vi "0 -5 Connect Message Display.vi"() -> ()   [LabVIEW 2012]
panel:
  out "Base + Entension Number":dbl
  in  "Base Number":dbl=1200.0 min=1000.0 step=10.0
  in  "OK Button":bool
  in  "Extension Number":dbl min=0.0 max=5.0 step=1.0
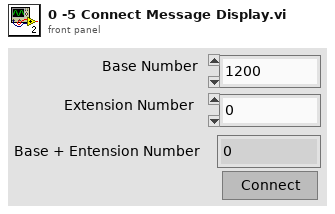
[diagram p1: front panel]
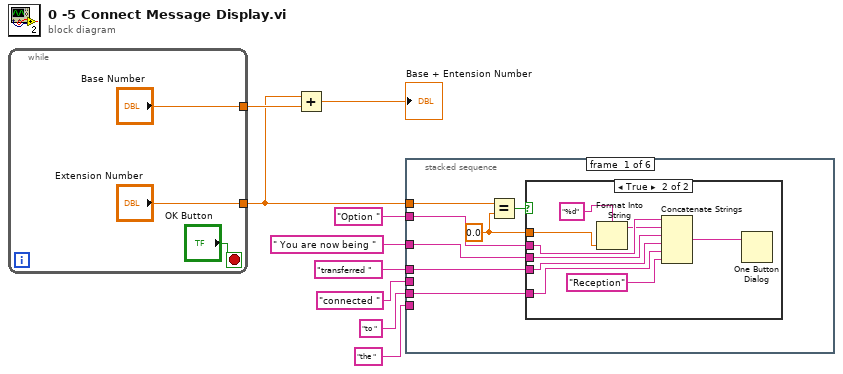
[diagram p0: block diagram]
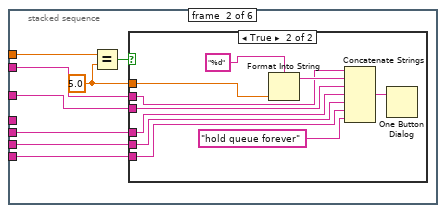
[diagram p3: hidden frame]
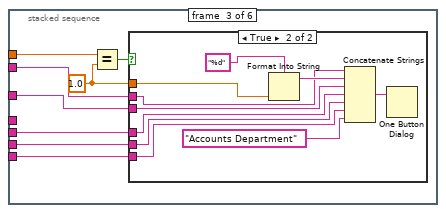
[diagram p5: hidden frame]
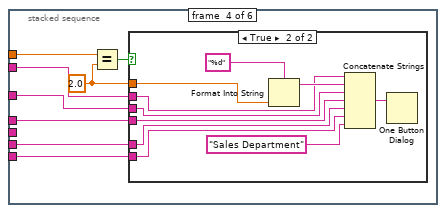
[diagram p7: hidden frame]
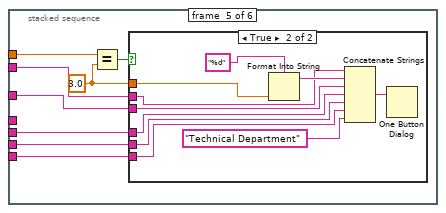
[diagram p9: hidden frame]
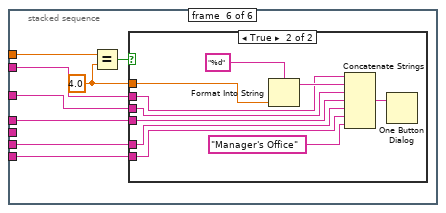
[diagram p11: hidden frame]
diagram:
  n1 = while {
    tunnel: ["Extension Number"] -> w1
    tunnel: ["Base Number"] -> w2
    stop <- "OK Button" stop-if-true
  }
  n2 = Add(x=w1, y=w2) -> (x+y=→"Base + Entension Number":dbl)
  n3 = stacked-sequence {
    tunnel: "Option " -> [w18 w30 w52 w70 w88 w105]
    tunnel: " You are now being " -> [w17 w31 w51 w69 w87 w104]
    tunnel: "transferred " -> [w16 _ _ w67 _ w103]
    tunnel: "to " -> [w15 w34 w49 w66 w83 w102]
    tunnel: w1 -> [w13 w29 w54 w68 w86 w106]
    tunnel: "connected " -> [_ w32 w50 _ w84 _]
    tunnel: "the " -> [_ w33 w48 w65 w85 w101]
    frame #0 {
      w14 = 0.0
      n4 = Equal?(x=w13, y=w14) -> (x = y?=w19:bool)
      n5 = case shown="True" w19 {
        tunnel: w18 -> [_ w28]
        tunnel: w17 -> [_ w26]
        tunnel: w16 -> [_ w25]
        tunnel: w15 -> [_ w24]
        tunnel: w14 -> [_ w22]
        frame False {
        }
        frame True {
          n6 = Format Into String(format string="%d", w22) -> (resulting string=w21:string)  [unwired: 2 in, 1 out]
          n7 = Concatenate Strings(w28, w21, w26, w25, w24, "Reception") -> (w27:string)
          n8 = One Button Dialog(message=w27) -> ()  [unwired: 1 in, 1 out]
        }
      }
    }
    frame #1 {
      w36 = 5.0
      n9 = Equal?(x=w29, y=w36) -> (x = y?=w35:bool)
      n10 = case shown="True" w35 {
        tunnel: w36 -> [_ w44]
        tunnel: w30 -> [_ w43]
        tunnel: w31 -> [_ w42]
        tunnel: w32 -> [_ w41]
        tunnel: w34 -> [_ w40]
        tunnel: w33 -> [_ w39]
        frame False {
        }
        frame True {
          n11 = Format Into String(format string="%d", w44) -> (resulting string=w45:string)  [unwired: 2 in, 1 out]
          n12 = Concatenate Strings(w43, w45, w42, w41, w40, w39, "hold queue forever") -> (w46:string)
          n13 = One Button Dialog(message=w46) -> ()  [unwired: 1 in, 1 out]
        }
      }
    }
    frame #2 {
      w53 = 1.0
      n14 = Equal?(x=w54, y=w53) -> (x = y?=w47:bool)
      n15 = case shown="True" w47 {
        tunnel: w53 -> [_ w62]
        tunnel: w52 -> [_ w61]
        tunnel: w51 -> [_ w60]
        tunnel: w50 -> [_ w59]
        tunnel: w49 -> [_ w58]
        tunnel: w48 -> [_ w57]
        frame False {
        }
        frame True {
          n16 = Format Into String(format string="%d", w62) -> (resulting string=w63:string)  [unwired: 2 in, 1 out]
          n17 = Concatenate Strings(w61, w63, w60, w59, w58, w57, "Accounts Department") -> (w64:string)
          n18 = One Button Dialog(message=w64) -> ()  [unwired: 1 in, 1 out]
        }
      }
    }
    frame #3 {
      w71 = 2.0
      n19 = Equal?(x=w68, y=w71) -> (x = y?=w72:bool)
      n20 = case shown="True" w72 {
        tunnel: w71 -> [_ w80]
        tunnel: w70 -> [_ w79]
        tunnel: w69 -> [_ w78]
        tunnel: w66 -> [_ w77]
        tunnel: w65 -> [_ w76]
        tunnel: w67 -> [_ w73]
        frame False {
        }
        frame True {
          n21 = Format Into String(format string="%d", w80) -> (resulting string=w81:string)  [unwired: 2 in, 1 out]
          n22 = Concatenate Strings(w79, w81, w78, w73, w77, w76, "Sales Department") -> (w82:string)
          n23 = One Button Dialog(message=w82) -> ()  [unwired: 1 in, 1 out]
        }
      }
    }
    frame #4 {
      w90 = 3.0
      n24 = Equal?(x=w86, y=w90) -> (x = y?=w89:bool)
      n25 = case shown="True" w89 {
        tunnel: w90 -> [_ w98]
        tunnel: w88 -> [_ w97]
        tunnel: w87 -> [_ w96]
        tunnel: w84 -> [_ w95]
        tunnel: w83 -> [_ w94]
        tunnel: w85 -> [_ w93]
        frame False {
        }
        frame True {
          n26 = Format Into String(format string="%d", w98) -> (resulting string=w99:string)  [unwired: 2 in, 1 out]
          n27 = Concatenate Strings(w97, w99, w96, w95, w94, w93, "Technical Department") -> (w100:string)
          n28 = One Button Dialog(message=w100) -> ()  [unwired: 1 in, 1 out]
        }
      }
    }
    frame #5 {
      w108 = 4.0
      n29 = Equal?(x=w106, y=w108) -> (x = y?=w107:bool)
      n30 = case shown="True" w107 {
        tunnel: w108 -> [_ w116]
        tunnel: w105 -> [_ w115]
        tunnel: w104 -> [_ w114]
        tunnel: w103 -> [_ w113]
        tunnel: w102 -> [_ w112]
        tunnel: w101 -> [_ w109]
        frame False {
        }
        frame True {
          n31 = Format Into String(format string="%d", w116) -> (resulting string=w117:string)  [unwired: 2 in, 1 out]
          n32 = Concatenate Strings(w115, w117, w114, w113, w112, w109, "Manager's Office") -> (w118:string)
          n33 = One Button Dialog(message=w118) -> ()  [unwired: 1 in, 1 out]
        }
      }
    }
  }
